vi "写入固件.vi"(8 "错误输入":errorcluster, 11 "MB session in":refnum<class "MB_Master.lvclass">) -> (0 "error out":errorcluster, 3 "MB session out":refnum<class "MB_Master.lvclass">)   [LabVIEW 2016, in "斯坦道总氮.lvlib"]
uses:
  <vilib>/Plasmionique/MB Master/MB_Master/MB_Master.lvclass
  <vilib>/NI/Progress Bar/Controls/Update Bar Actions.ctl
  <vilib>/NI/Progress Bar/Controls/Progress Bar Properties.ctl
  <vilib>/Plasmionique/MB Master/MB_Master_Serial/MB_Master_Serial.lvclass
  C:/Program Files (x86)/National Instruments/LabVIEW 2016/vi.lib/Plasmionique/MB Master/MB_Master/MB_Master.lvclass
  <vilib>/Plasmionique/MB Master/MB Master.lvlib
  <vilib>/NI/Progress Bar/Progress Bar.lvlib
panel:
  in  "引用选择":enum16{"MB引用", "自建引用"}(ring)
  in  "VISA Resource":refnum<visa-resource-name>
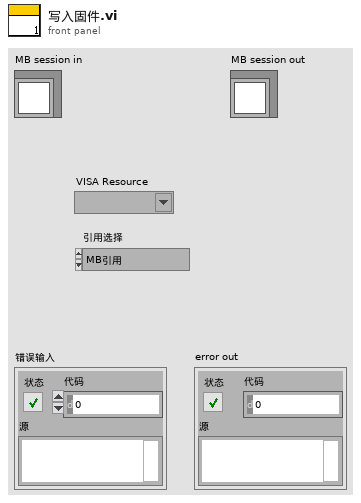
[diagram p1: front panel]
types:
  T1 = enum16{"open", "replace", "create", "open or create", "replace or create", "replace or create with confirmation"}
  T2 = enum16{"big-endian, network order", "native, host order", "little-endian"}
  T3 = typedef "Progress Bar.lvlib/Update Bar Actions.ctl" = enum16{"Add To Existing", "Set to Value"}
  T4 = cluster{"baud rate (bps)":u32, "stop bits":u16, "parity":u16, "flow control":u16, "timeout":u32, "retries":i32}
  T5 = typedef "Progress Bar.lvlib/Progress Bar Properties.ctl" = cluster{"Background Color":u32, "Installer Title":string, "Title Color":u32, "Action Text":string, "Text Color":u32, "Slider Value":u8, "Bar Color":u32, "Timeout":i32}
  T6 = cluster{"泵类型":u8, "进样速度":u32, "出样速度":u32, "泵阀量":u8, "光谱仪类型":u8, "光谱采样次数":u8, "氙灯次数":u8, "B":u16, "C":u16, "D":u16, "E":u16, "B_COD":u16, "C_COD":u16, "D_COD":u16, "E_COD":u16, "G":u16, "M":u16, "N":u16, "氨氮注射泵控温下限":sgl, "氨氮注射泵控温上限":sgl, "总氮注射泵控温下限":sgl, "总氮注射泵控温上限":sgl, "消解温度下限":sgl, "消解温度上限":sgl, "加热10s限值":sgl, "高温高压阀开阀温度":sgl, "总氮x公式0":u8, "总氮x公式1":sgl, "总氮x公式2":sgl, "总磷浊度稀释系数":sgl, "总磷浊度补偿权重1":sgl, "总磷浊度补偿权重2":sgl, "盐度系数":sgl, "氨氮补偿系数1":sgl, "氨氮补偿系数2":sgl}
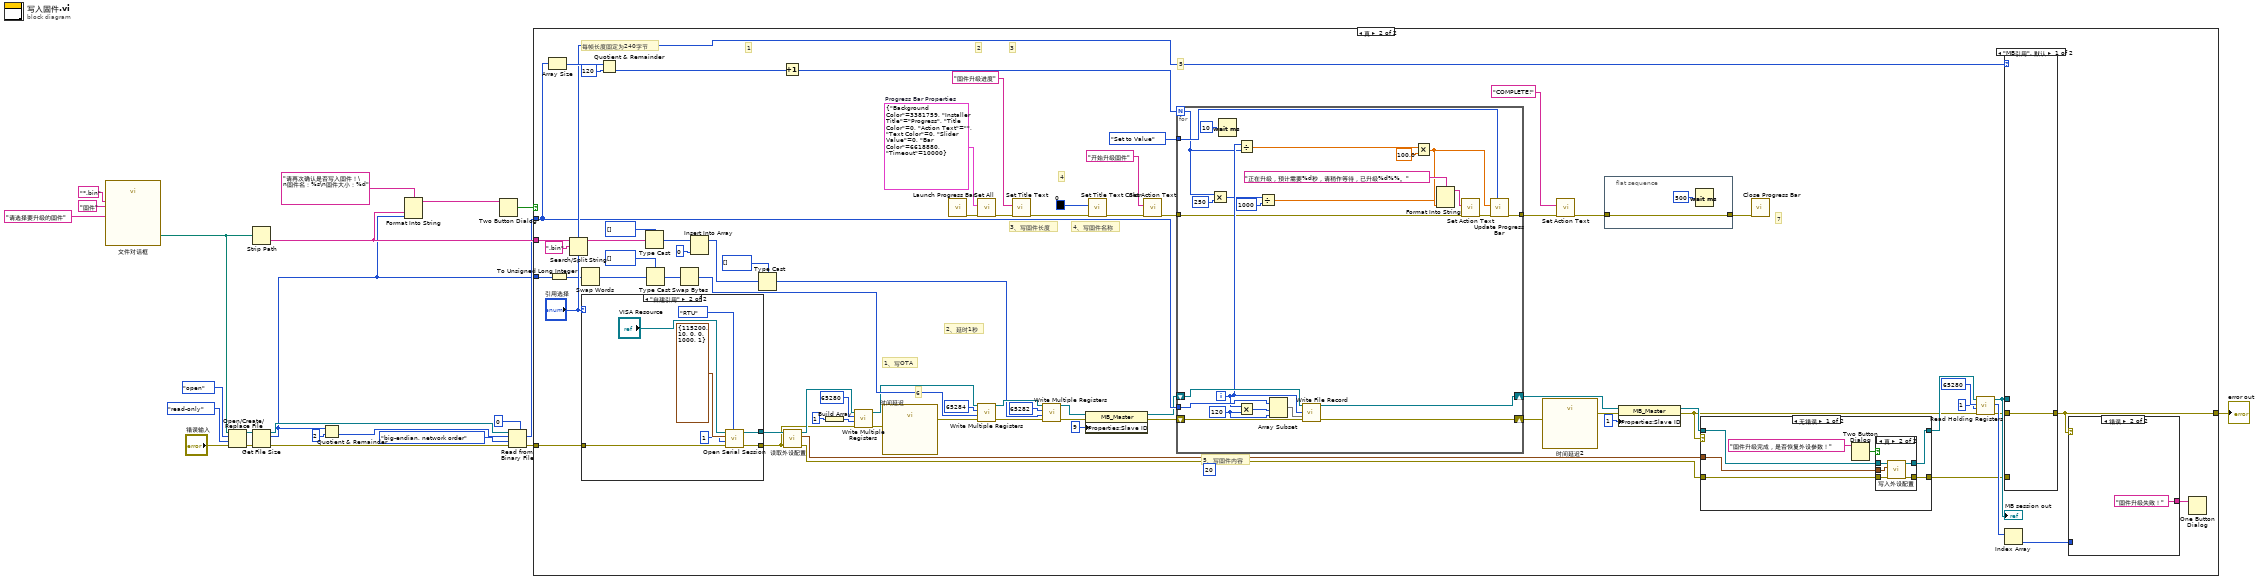
[diagram p0: block diagram]
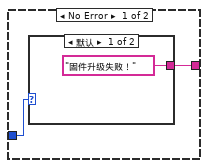
[diagram p5: hidden frame]
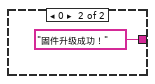
[diagram p6: hidden frame]
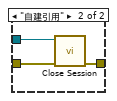
[diagram p7: hidden frame]
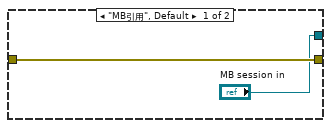
[diagram p8: hidden frame]
diagram:
  n1 = call "文件对话框"("prompt"="请选择要升级的固件", "pattern (all files)"="*.bin", "pattern label"="固件") -> ("selected path"=w10:path)  [unwired: 9 in, 3 out]
  n2 = Open/Create/Replace File(file path (use dialog)=w10, error in="错误输入", operation (0:open)=T1."open" ("操作(0:open)"), access (0:read/write)=enum16{"read/write", "read-only", "write-only"}."read-only" ("权限(0:read/write)")) -> (refnum out=w9:refnum<file>, error out=w7:errorcluster)  [unwired: 2 in, 1 out]
  n3 = Strip Path(path=w10) -> (name=w18:string)  [unwired: 1 out]
  n4 = Get File Size(file=w9, error in=w7) -> (refnum out=w8:refnum<file>, size (in bytes)=w2:i64, 0:w6:errorcluster)
  n5 = Quotient & Remainder(x=w2, y=i64 2) -> (floor(x/y)=w4:i64)  [unwired: 1 out]
  n6 = Format Into String(format string="请再次确认是否写入固件！\n固件名：%s\n固件大小：%d" ("格式字符串"), w18, w2) -> (resulting string=w17:string)  [unwired: 2 in, 1 out]
  n7 = Two Button Dialog(message=w17) -> (T button?=w16:bool)  [unwired: 2 in]
  n8 = Read from Binary File(5:u16 0, 8:w6, 9:T2."big-endian, network order" ("字节顺序(0:big-endian, network order)"), 10:w4, 11:w8) -> (0:w15:errorcluster, 2:w3:u16[])  [unwired: 1 in, 2 out]
  n9 = case shown="真" w16 {
    tunnel: w3 -> [_ w61]
    tunnel: w18 -> [_ w77]
    tunnel: w15 -> [w24 w79]
    tunnel: [w24 w49] -> w13
    tunnel: w2 -> [_ w63]
    frame False {
    }
    frame True {
      w46 = T5 {"Background Color"=3381759, "Installer Title"="Progress", "Title Color"=0, "Action Text"="", "Text Color"=0, "Slider Value"=0, "Bar Color"=6618880, "Timeout"=10000}  # Progress Bar Properties
      (unwired) 20 ("Value")
      # "7"
      # "6"
      # "5"
      # "4"
      # "3"
      # "2"
      # "1"
      # "每帧长度固定为240字节"
      # "5、写固件内容"
      # "4、写固件名称"
      # "3、写固件长度"
      # "2、延时1秒"
      # "1、写OTA"
      n10 = Array Size(array=w61) -> (size(s)=w95:i32)
      n11 = To Unsigned Long Integer(number=w63) -> (unsigned 32bit integer=w55:u32)
      n12 = Search/Split String(string=w77, search string/char (-)=".bin" ("搜索字符串/字符(-)")) -> (substring before match=w75:string)  [unwired: 1 in, 2 out]
      n13 = Swap Words(1:w55) -> (0:w54:u32)
      n14 = case shown="\"自建引用\"" "引用选择" {
        tunnel: ["MB session in" w131] -> w80
        tunnel: w79 -> [w125 w130]
        tunnel: [w125 w129] -> w29
        frame "MB引用", Default {
        }
        frame "自建引用" {
          n15 = call <vilib>:"Open Serial Session.vi"("Mode (RTU)"=enum16{"RTU", "ASCII"}."RTU", "Error in"=w130, "Slave ID"=u8 1, "Serial Config"=T4 {"baud rate (bps)"=115200, "stop bits"=10, "parity"=0, "flow control"=0, "timeout"=1000, "retries"=1}, "VISA Resource"="VISA Resource") -> ("Error out"=w129:errorcluster, "MB_Serial session"=w131:refnum<class "MB_Master_Serial.lvclass">)  [unwired: 5 in]
        }
      }
      n16 = Quotient & Remainder(x=w95, y=120) -> (floor(x/y)=w96:i32)  [unwired: 1 out]
      n17 = Type Cast(type=u8[] [], x=w75) -> (*(type *) &x=w83:u8[])
      n18 = Type Cast(type=u16[] [], x=w54) -> (*(type *) &x=w89:u16[])
      n19 = Swap Bytes(anything=w89) -> (byte swapped=w88:u16[])
      n20 = Insert Into Array(array=w83, new element=u8 0 ("新元素/子数组")) -> (w74:u8[])  [unwired: 1 in]
      n21 = Type Cast(type=u16[] [], x=w74) -> (*(type *) &x=w73:u16[])
      n22 = Increment(x=w96) -> (x+1=w62:i32)
      n23 = call "读取外设配置.vi"("error in (no error)"=w29, "MB session in"=w80) -> ("error out"=w28:errorcluster, "外设配置"=w26:T6, "MB session out"=w31:refnum<class "MB_Master.lvclass">)  [unwired: 7 in]
      n24 = Build Array(u16 1 ("value")) -> (w81:u16[])
      n25 = call <vilib>:"Write Multiple Registers.vi"("error in (no error)"=w29, "values"=w81, "starting address"=u16 65280, "MB session in"=w31) -> ("error out"=w91:errorcluster, "MB session out"=w66:refnum<class "MB_Master.lvclass">)  [unwired: 6 in]
      n26 = call "时间延迟"("error in (no error)"=w91) -> ("error out"=w67:errorcluster)  [unwired: 10 in]
      n27 = call <vilib>:"Launch Progress Bar.vi"() -> ("error out"=w45:errorcluster)  [unwired: 10 in, 1 out]
      n28 = call <vilib>:"Set All.vi"("error in (no error)"=w45, "Progress Bar Properties (Default)"=w46) -> ("error out"=w39:errorcluster)  [unwired: 9 in]
      n29 = call <vilib>:"Write Multiple Registers.vi"("error in (no error)"=w67, "values"=w88, "starting address"=u16 65284, "MB session in"=w66) -> ("error out"=w86:errorcluster, "MB session out"=w87:refnum<class "MB_Master.lvclass">)  [unwired: 6 in]
      n30 = call <vilib>:"Set Title Text.vi"("error in (no error)"=w39, "Installer Title"="固件升级进度") -> ("error out"=w37:errorcluster)  [unwired: 9 in]
      n31 = call <vilib>:"Write Multiple Registers.vi"("error in (no error)"=w86, "values"=w73, "starting address"=u16 65282, "MB session in"=w87) -> ("error out"=w57:errorcluster, "MB session out"=w60:refnum<class "MB_Master.lvclass">)  [unwired: 6 in]
      n32 = property class="MB_Master"(reference=w60, error in=w57, "Properties:Slave ID"=u8 9 ("Slave ID")) -> (reference out=w58:refnum<class "MB_Master.lvclass">, error out=w56:errorcluster)
      n33 = call <vilib>:"Set Title Text Color.vi"("error in (no error)"=w37, "Color Box"=u32 0) -> ("error out"=w40:errorcluster)  [unwired: 9 in]
      n34 = call <vilib>:"Set Action Text.vi"("error in (no error)"=w40, "Action Text"="开始升级固件") -> ("error out"=w34:errorcluster)  [unwired: 9 in]
      n35 = for {
        N: w62 -> [w134]
        shift-right: [w154] -> w53
        shift-left: w58 -> [w156]
        shift-right: [w152] -> w51
        shift-left: w56 -> [w155]
        tunnel: w61 -> [w151]
        tunnel: Update_Bar_Actions."Set to Value" ("Action") -> [w146]
        tunnel: w34 -> [w144]
        tunnel: [w145] -> w33
        i -> [w149]
        w148 = 120 ("长度")
        n36 = Multiply(x=w134, y=250) -> (x*y=w138:i32)
        n37 = Wait (ms)(milliseconds to wait=u32 10) -> ()  [unwired: 1 out]
        n38 = Divide(x=w149, y=w134) -> (x/y=w140:dbl)
        n39 = Multiply(x=w149, y=w148) -> (x*y=w147:i32)
        n40 = Divide(x=w138, y=u32 1000) -> (x/y=w135:dbl)
        n41 = Array Subset(array=w151, index=w147, length=w148) -> (w150:u16[])
        n42 = call "Write File Record.vi"("MB session in"=w156, "Record Number"=w149, "values"=w150, "error in (no error)"=w155) -> ("MB session out"=w154:refnum<class "MB_Master.lvclass">, "error out"=w152:errorcluster)  [unwired: 10 in]
        n43 = Multiply(x=w140, y=100.0) -> (x*y=w136:dbl)
        n44 = Format Into String(format string="正在升级，预计需要%d秒，请稍作等待，已升级%d%%。" ("格式字符串"), w135, w136) -> (resulting string=w141:string)  [unwired: 2 in, 1 out]
        n45 = call <vilib>:"Set Action Text.vi"("error in (no error)"=w144, "Action Text"=w141) -> ("error out"=w143:errorcluster)  [unwired: 9 in]
        n46 = call <vilib>:"Update Progress Bar.vi"("Action"=w146, "error in (no error)"=w143, "Value"=w136) -> ("error out"=w145:errorcluster)  [unwired: 8 in]
      }
      n47 = call "时间延迟2"("error in (no error)"=w51) -> ("error out"=w32:errorcluster)  [unwired: 10 in]
      n48 = call <vilib>:"Set Action Text.vi"("error in (no error)"=w33, "Action Text"="COMPLETE!") -> ("error out"=w42:errorcluster)  [unwired: 9 in]
      n49 = flat-sequence {
        tunnel: w42 -> [w113]
        tunnel: [w113] -> w44
        frame #0 {
          n50 = Wait (ms)(milliseconds to wait=u32 500) -> ()  [unwired: 1 out]
        }
      }
      n51 = property class="MB_Master"(reference=w53, error in=w32, "Properties:Slave ID"=u8 1 ("Slave ID")) -> (reference out=w52:refnum<class "MB_Master.lvclass">, error out=w25:errorcluster)
      n52 = case shown="无错误" w25 {
        tunnel: w52 -> [w103 w112]
        tunnel: [w102 w112] -> w30
        tunnel: w28 -> [w101 w111]
        tunnel: [w100 w111] -> w27
        tunnel: w26 -> [w99 _]
        frame No Error {
          n53 = Two Button Dialog(message="固件升级完成，是否恢复外设参数！" ("消息")) -> (T button?=w97:bool)  [unwired: 2 in]
          n54 = case shown="真" w97 {
            tunnel: w103 -> [w105 w110]
            tunnel: [w105 w109] -> w102
            tunnel: w101 -> [w104 w108]
            tunnel: [w104 w107] -> w100
            tunnel: w99 -> [_ w106]
            frame False {
            }
            frame True {
              n55 = call "写入外设配置.vi"("error in (no error)"=w108, "外设配置"=w106, "MB session in"=w110) -> ("error out"=w107:errorcluster, "MB session out"=w109:refnum<class "MB_Master.lvclass">)  [unwired: 7 in]
            }
          }
        }
        frame Error {
        }
      }
      n56 = call <vilib>:"Close Progress Bar.vi"("error in (no error)"=w44) -> ()  [unwired: 9 in, 2 out]
      n57 = call <vilib>:"Read Holding Registers.vi"("error in (no error)"=w25, "quantity"=u16 1, "starting address"=u16 65280, "MB session in"=w30) -> ("error out"=w64:errorcluster, "Registers"=w68:u16[], "MB session out"=w65:refnum<class "MB_Master.lvclass">)  [unwired: 5 in]
      "MB session out" <- w65
      n58 = case shown="\"MB引用\", 默认" "引用选择" {
        tunnel: w65 -> [_ w123]
        tunnel: w64 -> [w120 w122]
        tunnel: [w120 w121] -> w49
        tunnel: w27 -> [_ _]
        frame "MB引用", Default {
        }
        frame "自建引用" {
          n59 = call-dynamic "Close Session.vi"("error in (no error)"=w122, "MB session in"=w123) -> ("error out"=w121:errorcluster)  [unwired: 9 in]
        }
      }
      n60 = Index Array(array=w68) -> (element=w48:u16)  [unwired: 1 in]
      n61 = case shown="错误" w49 {
        tunnel: w48 -> [w116 _]
        tunnel: [w115 "固件升级失败！"] -> w47
        frame No Error {
          n62 = case shown="默认" w116 {
            tunnel: ["固件升级失败！" "固件升级成功！"] -> w115
            frame Default {
            }
            frame 0 {
            }
          }
        }
        frame Error {
        }
      }
      n63 = One Button Dialog(message=w47) -> ()  [unwired: 1 in, 1 out]
    }
  }
  "error out" <- w13
